vi "Fetch Multiple Record Single Channel (Wfm).vi"(5 "FIFO Type":enum16{"FPGA to Host FIFO (U64)", "Generic"}(ring), 7 "Timeout (s)":i32=5, 8 "error in":errorcluster, 10 "Records to Fetch":i32, 11 "FPGA VI Reference In":refnum<k20>) -> (0 "error out":errorcluster, 2 "Acquire Data":waveform(dbl)[](array[waveform]), 3 "FPGA VI Reference Out":refnum<k20>, 4 "Elements Remaining":u32)   [LabVIEW 2011]
uses:
  <userlib>/FlexRIO Host Library/FlexRIO Host API/Acquire/Fetch/Fetch Acquired Data (U64).vi
  <vilib>/Utility/error.llb/Error Cluster From Error Code.vi
  <vilib>/rvi/errors/niLvFpgaAdjustHostInterfaceError.vi
  <vilib>/rvi/interface/nirviReadWriteControl/nirviReadWriteControl.xnode
  NiFpgaLv.dll
  <vilib>/rvi/interface/Simulation/niFpgaSimulationCallBeginRW.vi
  <userlib>/FlexRIO Host Library/FlexRIO Host Library (User).lvlib
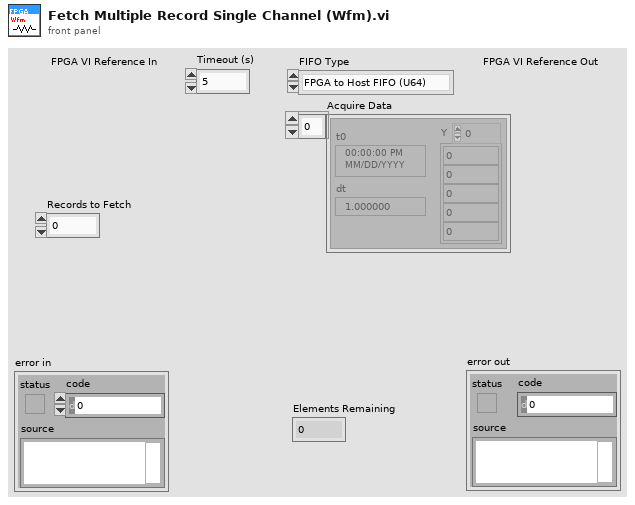
[diagram p1: front panel]
types:
  T1 = cluster{"Load Record Parameters?":bool, "Pre Trigger Samples":u16, "Samples per Record":u16, "Trigger Hold Off":u16, "Record Count":u16}
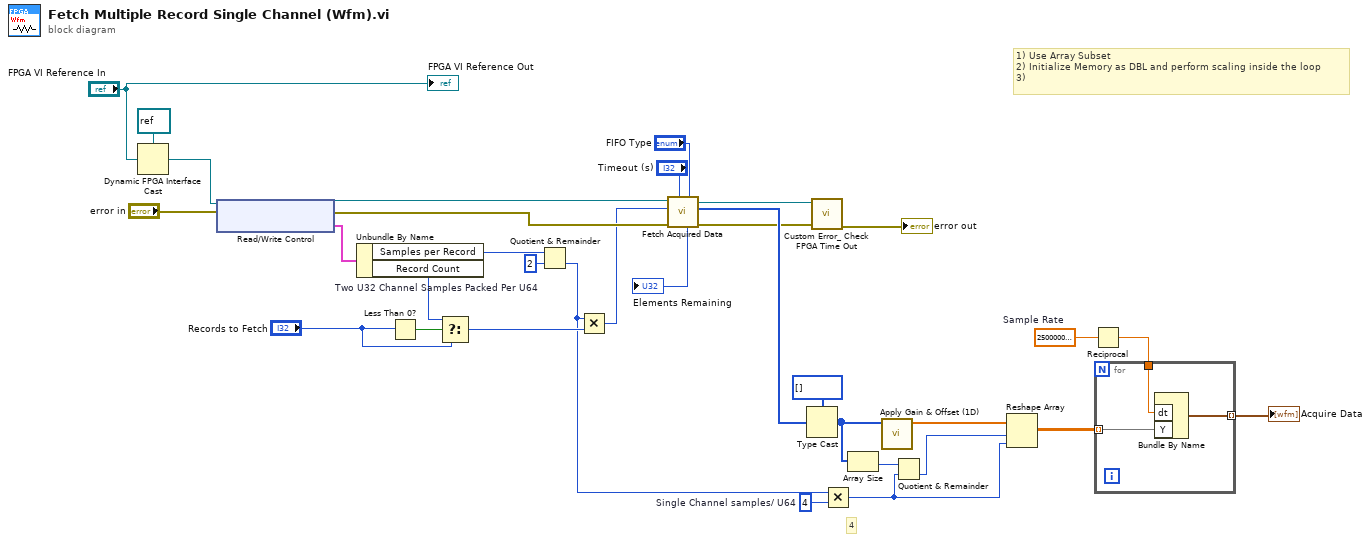
[diagram p0: block diagram]
diagram:
  w2 = 250000000.0  # Sample Rate
  w7 = u16 2  # Two U32 Channel Samples Packed Per U64
  w17 = u16 4  # Single Channel samples/ U64
  # "4"
  # "1) Use Array Subset\n2) Initialize Memory as DBL and perform scaling inside the loop\n3)"
  n1 = Dynamic FPGA Interface Cast(Session In=refnum<k20> refnum ("Type"), Type="FPGA VI Reference In") -> (Session Out=w30:refnum<k20>)
  n2 = xnode "Read/Write Control"("FPGA VI Reference In"=w30, "error in"="error in") -> ("FPGA VI Reference Out"=w25:refnum<k20>, "error out"=w24:errorcluster, "Record Parameters"=w29:T1)
  n3 = Unbundle By Name(w29) -> ("Samples per Record"=w8:u16, "Record Count"=w27:u16)
  n4 = Less Than 0?(x="Records to Fetch") -> (x < 0?=w28:bool)
  n5 = Select(t=w27, s=w28, f="Records to Fetch") -> (s? t:f=w18:i32)
  n6 = Quotient & Remainder(x=w8, y=w7) -> (floor(x/y)=w9:u16)  [unwired: 1 out]
  n7 = Multiply(x=w9, y=w18) -> (x*y=w13:i32)
  n8 = call-poly <userlib>:"Fetch Acquired Data.vi"("FIFO Type"="FIFO Type", "Timeout (s)"="Timeout (s)", "error out"=w24, "Samples"=w13, "FPGA VI Reference In"=w25) -> ("error out"=w15:errorcluster, "Data"=w21:u64[], "FPGA VI Reference Out"=w16:refnum<k20>, "Elements Remaining"=→"Elements Remaining":u32)  [unwired: 3 in]
  n9 = Type Cast(type=i16[] [], x=w21) -> (*(type *) &x=w6:i16[])
  n10 = call <userlib>:"Custom Error_ Check FPGA Time Out.vi"("error in"=w15, "FPGA VI Reference In"=w16) -> ("error out"=→"error out":errorcluster)  [unwired: 8 in, 1 out]
  n11 = Multiply(x=w9, y=w17) -> (x*y=w11:u16)
  n12 = Array Size(array=w6) -> (size(s)=w12:i32)
  n13 = call <userlib>:"Apply Gain & Offset (1D).vi"("Raw Data"=w6) -> ("Scaled Data"=w5:dbl[])  [unwired: 10 in]
  n14 = Quotient & Remainder(x=w12, y=w11) -> (floor(x/y)=w10:i32)  [unwired: 1 out]
  n15 = Reshape Array(w5, w10, w11) -> (w4:dbl[][])
  n16 = Reciprocal(x=w2) -> (1/x=w1:dbl)
  n17 = for {
    tunnel: w4 -> [w34] mode=indexing
    tunnel: [w36] -> w3 mode=indexing
    tunnel: w1 -> [w35]
    n18 = Bundle By Name("dt"=w35, "Y"=w34) -> (w36:waveform(dbl))  [unwired: 1 in]
  }
  "Acquire Data" <- w3
  "FPGA VI Reference Out" <- "FPGA VI Reference In"
